vi "display loop backup.vi"(0 "display queues":T4, 3 "time range (s)":dbl=2.2 format="%#_13g", 4 "mag type":enum16{"absolute", "relative"}(ring), 5 "volt slope":bool, 7 "error in":errorcluster, 8 "trigger":bool, 9 "hysteresis":dbl=0.1 format="%#_13g", 10 "disk queues":T4, 11 "L/z0":dbl format="%#_13g", 12 "gain":dbl=1.0) -> (16 "magnet vs time":cluster{dbl[], dbl[]}[](array[cluster]), 17 "mag pos axes limits":cluster{"mag pos max":dbl, "mag pos min":dbl}, 18 "voltage axes":T1, 19 "crossing stats":T2, 20 "fit parameters":T3, 23 "fit time":u32, 24 "fitter error":bool, 25 "voltage graphs":cluster{dbl[], dbl[]}[](array[cluster]), 26 "magnet graphs":T6(array[cluster]), 27 "error out":errorcluster)   [LabVIEW 2017]
uses:
  popup panels/control panel globals.vi
  typedefs/queue cluster.ctl
  typedefs/readingType.ctl
  typedefs/reading.ctl
  typedefs/reading queue.ctl
  typedefs/magnetic field fit.ctl
  typedefs/magnetomter reading set.ctl
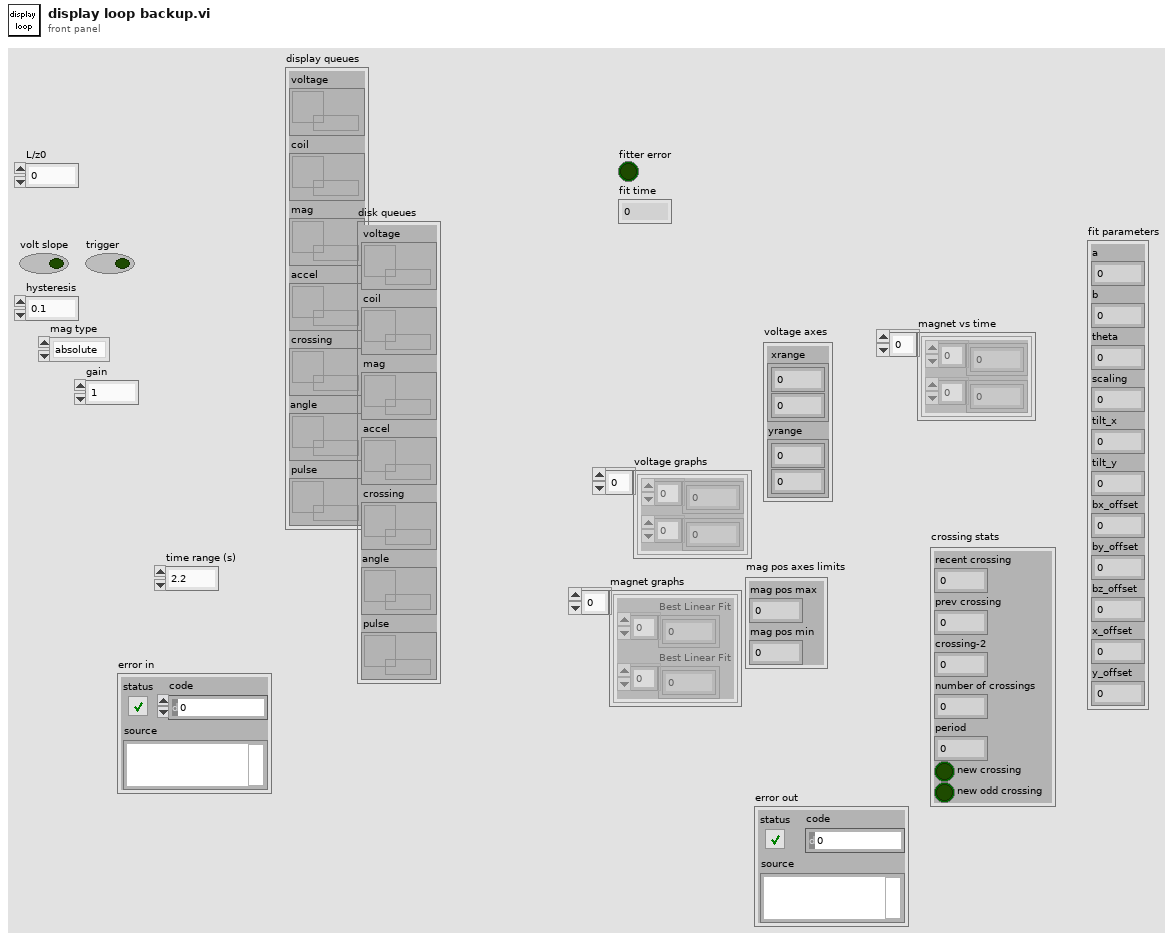
[diagram p1: front panel]
types:
  T1 = cluster{" xrange":cluster{dbl, dbl}, "yrange":cluster{dbl, dbl}}
  T2 = cluster{"recent crossing":dbl, "prev crossing":dbl, "crossing-2":dbl, "number of crossings":i32, "period":dbl, "new crossing":bool, "new odd crossing":bool}
  T3 = typedef "magnetic field fit.ctl" = cluster{"a":dbl, "b":dbl, "theta":dbl, "scaling":dbl, "tilt_x":dbl, "tilt_y":dbl, "bx_offset":dbl, "by_offset":dbl, "bz_offset":dbl, "x_offset":dbl, "y_offset":dbl}
  T4 = typedef "queue cluster.ctl" = cluster{"voltage":T5, "coil":T5, "mag":refnum<queue>, "accel":T5, "crossing":T5, "angle":T5, "pulse":T5}
  T5 = typedef "reading queue.ctl" = refnum<queue>
  T6 = cluster{"Best Linear Fit":dbl[], "Best Linear Fit":dbl[]}[]
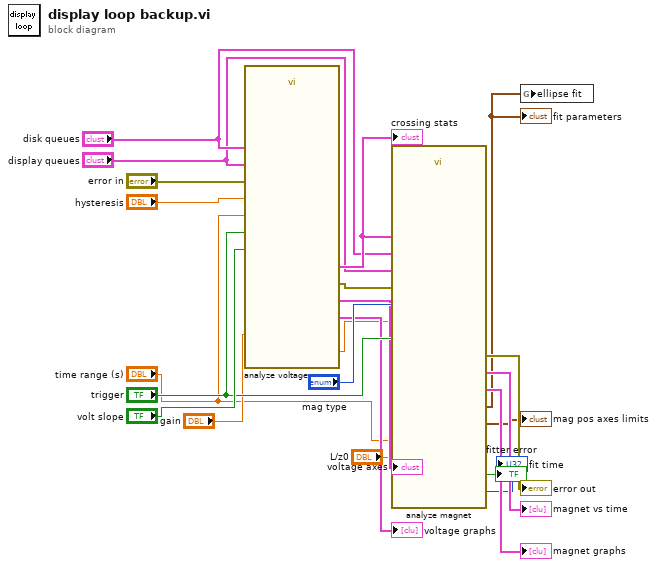
[diagram p0: block diagram]
diagram:
  n1 = call "analyze voltage.vi"("display queues"="display queues", "time range (s)"="time range (s)", "gain"="gain", "volt slope"="volt slope", "error in"="error in", "trigger"="trigger", "hysteresis"="hysteresis", "disk queues"="disk queues") -> ("crossing stats"=w19:T2, "t offset out"=w4:dbl, "voltage axes"=→"voltage axes":T1, "voltage graphs"=→"voltage graphs":cluster{dbl[], dbl[]}[], "error out"=w16:errorcluster)  [unwired: 15 in]
  "crossing stats" <- w19
  n2 = call "analyze magnet.vi"("display queues"="display queues", "disk queues"="disk queues", "time range (s)"="time range (s)", "trigger"="trigger", "graph type"="mag type", "error in (no error)"=w16, "L/z0"="L/z0", "toffset"=w4, "crossing stats"=w19) -> ("mag pos axes limits"=→"mag pos axes limits":cluster{"mag pos max":dbl, "mag pos min":dbl}, "x-y magnet graph"=→"magnet graphs":cluster{sgl[], sgl[]}[], "magnet time graphs"=→"magnet vs time":cluster{dbl[], sgl[]}[], "fit parameters"=w6:T3, "fitter error"=→"fitter error":bool, "fit time"=→"fit time":u32, "error out"=→"error out":errorcluster)  [unwired: 4 in]
  "fit parameters" <- w6
  n3 = global write "control panel globals.vi" "ellipse fit"(w6) -> ()
